vi "Iterative Max Value.vi"(11 "Array in":dbl[](array[numeric])) -> (1 "Array out":dbl[](array[numeric]), 2 "Max index":dbl, 3 "Max value":dbl)   [LabVIEW 2014, in "Aquisicao de Dados.lvlib"]
uses:
  Aquisicao de Dados.lvlib
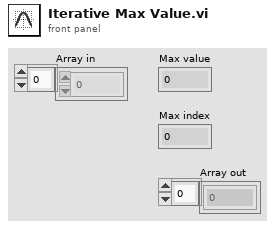
[diagram p1: front panel]
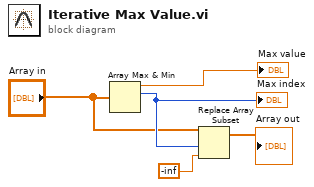
[diagram p0: block diagram]
diagram:
  n1 = Array Max & Min(array="Array in") -> (max value=→"Max value":dbl, max index (indices)=w4:i32)  [unwired: 2 out]
  "Max index" <- w4
  n2 = Replace Array Subset(array="Array in", new element=-inf, index=w4) -> (→"Array out":dbl[])
